vi "check_local_waveform_cache_for_files.vi"() -> ()   [LabVIEW 2013]
uses:
  <vilib>/Utility/miscctls.llb/LVPointTypeDef.ctl
  <userlib>/_OpenG.lib/file/file.llb/Strip Path Extension - Path__ogtk.vi
  <vilib>/addons/database/Connection.llb/Conn Execute.vi
  <vilib>/addons/database/Recordset.llb/Rec Fetch Recordset Data (R).vi
  <vilib>/addons/database/Recordset.llb/Rec Destroy - Connection.vi
  <vilib>/addons/database/_DB Variant To Data/Database Variant To Data.xnode
  <vilib>/addons/database/NI_Database_API.lvlib
panel:
  out "error out":errorcluster
  out "Number of files with no entry":i32
  out "No Database Entry":string[](array[string])
  in  "Run?":bool
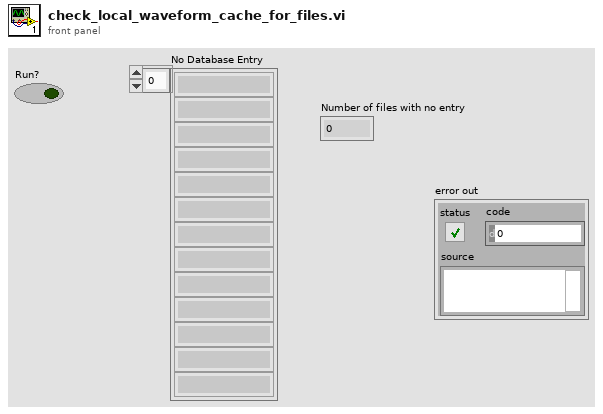
[diagram p1: front panel]
types:
  T1 = typedef "LVPointTypeDef.ctl" = cluster{"Horizontal":i16, "Vertical":i16}
  T2 = typedef "NI_Database_API.lvlib/Conn ObjectReference.ctl" = refnum<k1>
  T3 = typedef "NI_Database_API.lvlib/Rec ObjectReference.ctl" = refnum<k1>
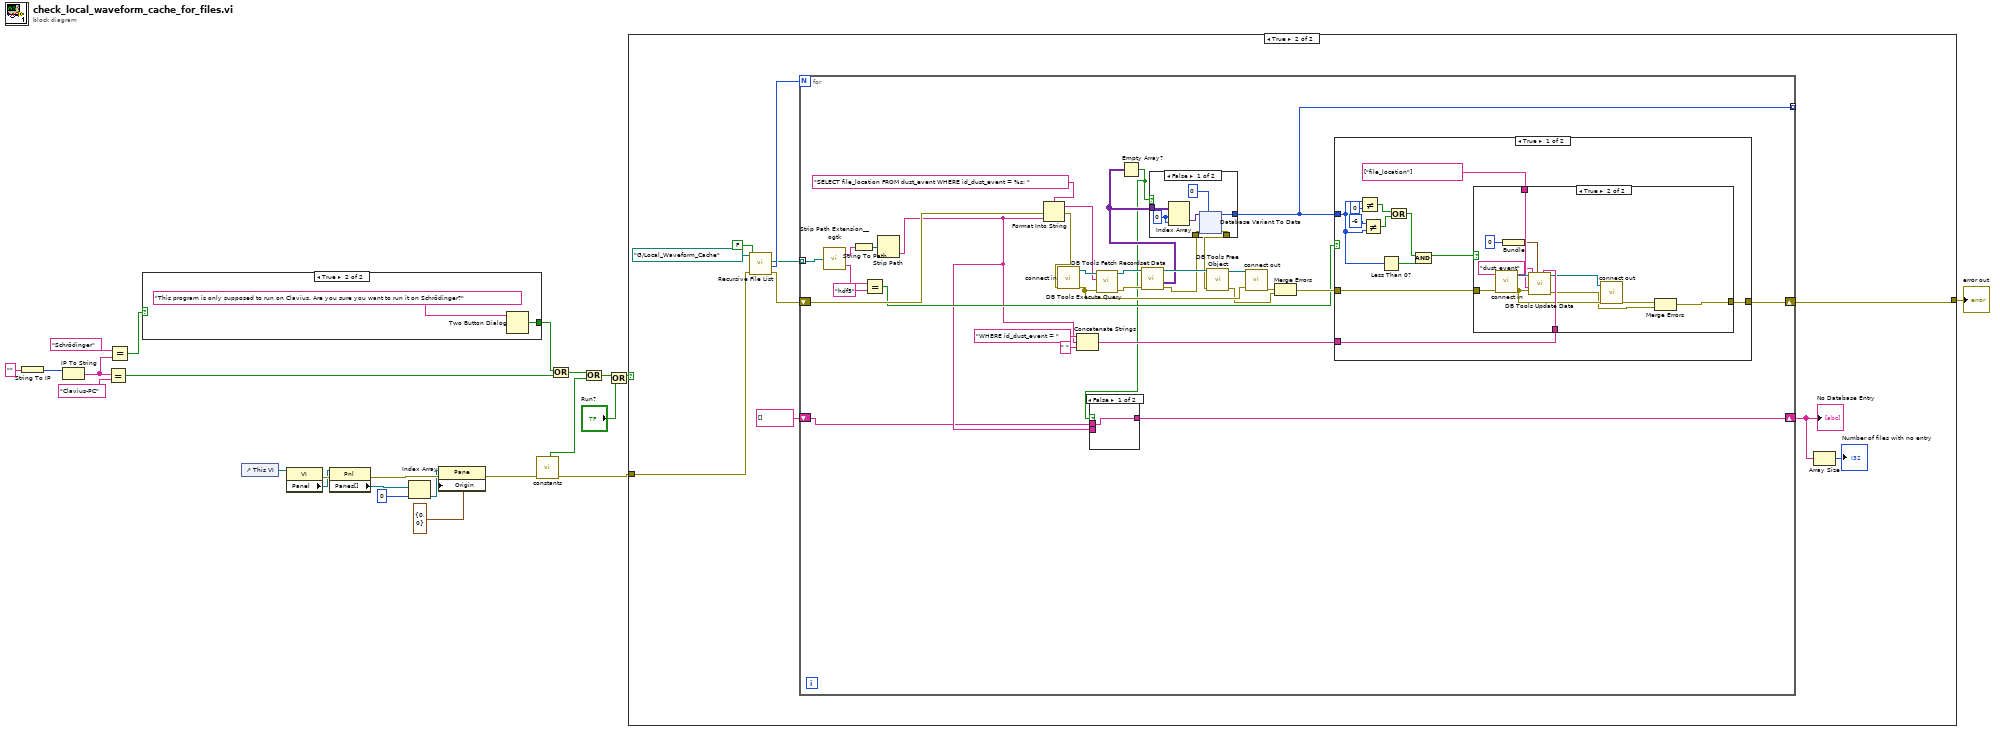
[diagram p0: block diagram]
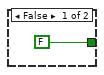
[diagram p2: hidden frame]
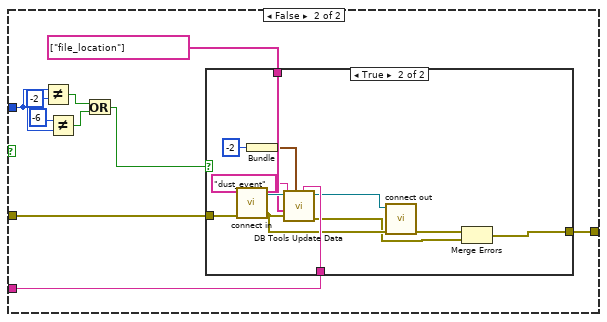
[diagram p5: hidden frame]
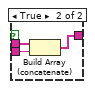
[diagram p7: hidden frame]
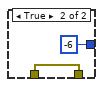
[diagram p8: hidden frame]
diagram:
  n1 = String To IP(1:"" ("name")) -> (0:w16:u32)
  n2 = IP To String(2:w16) -> (0:w11:string)  [unwired: 1 in]
  n3 = Equal?(x=w11, y="Clavius-PC") -> (x = y?=w8:bool)
  n4 = Equal?(x="Schrödinger", y=w11) -> (x = y?=w6:bool)
  n5 = case shown="True" w6 {
    tunnel: [FALSE ("T button?") w27] -> w7
    frame False {
    }
    frame True {
      n6 = Two Button Dialog(message="This program is only supposed to run on Clavius. Are you sure you want to run it on Schrödinger?") -> (T button?=w27:bool)  [unwired: 2 in]
    }
  }
  n7 = control-ref of="This VI"() -> (w24:refnum<vi>)
  n8 = property class="VI"(reference=w24) -> (error out=w23:errorcluster, "Panel"=w22:refnum<vi>)  [unwired: 1 in, 1 out]
  n9 = property class="Pnl"(reference=w22, error in=w23) -> (error out=w21:errorcluster, "Panes[]"=w20:refnum<vi>[])  [unwired: 1 out]
  n10 = Index Array(array=w20, index=0) -> (element=w18:refnum<vi>)
  n11 = property class="Pane"(reference=w18, error in=w21, "Origin"=T1 {"Horizontal"=0, "Vertical"=0}) -> (error out=w13:errorcluster)  [unwired: 1 out]
  n12 = call "constants.vi"("error in (no error)"=w13) -> ("error out"=w4:errorcluster, "Testing"=w12:bool)  [unwired: 4 in, 5 out]
  n13 = Or(x=w7, y=w8) -> (x .or. y?=w9:bool)
  n14 = Or(x=w9, y=w12) -> (x .or. y?=w5:bool)
  n15 = Or(x=w5, y="Run?") -> (x .or. y?=w3:bool)
  n16 = case shown="True" w3 {
    tunnel: w4 -> [w28 w36]
    tunnel: [w28 w29] -> w1
    frame False {
    }
    frame True {
      n17 = call <vilib>:"Recursive File List.vi"("error in (no error)"=w36, "Treat LLBs as Folders?"=FALSE, "Folder Path"=path "G:/Local_Waveform_Cache") -> ("error out"=w33:errorcluster, "Number of Files"=w35:i32, "All Files in Dir"=w34:path[])  [unwired: 4 in, 2 out]
      n18 = for {
        N: w35 -> [_]
        tunnel: w34 -> [w69] mode=indexing
        tunnel: [w45] -> _ mode=indexing
        shift-right: [w42] -> w31
        shift-left: string[] [] -> [w41]
        shift-right: [w39] -> w29
        shift-left: w33 -> [w64]
        n19 = call-poly <userlib>:"Strip Path Extension__ogtk.vi"("path"=w69) -> ("root"=w68:string, "extension"=w66:string)
        n20 = String To Path(string=w68) -> (path=w67:path)
        n21 = Equal?(x=w66, y="hdf5") -> (x = y?=w46:bool)
        n22 = Strip Path(path=w67) -> (name=w43:string)  [unwired: 1 out]
        n23 = Format Into String(format string="SELECT file_location FROM dust_event WHERE id_dust_event = %s; " ("SQL query"), error in=w64, w43) -> (resulting string=w58:string, error out=w59:errorcluster)  [unwired: 1 in]
        n24 = call "connect in.vi"("error in (no error)"=w59) -> ("error out"=w63:errorcluster, "Database Connection"=w61:T2)  [unwired: 6 in, 1 out]
        n25 = Concatenate Strings("WHERE id_dust_event = " ("string"), w43, " " ("string")) -> (w47:string)
        n26 = call-poly <vilib>:"DB Tools Execute Query.vi"("error in (no error)"=w63, "SQL query"=w58, "connection reference"=w61) -> ("error out"=w62:errorcluster, "recordset reference"=w57:T3)  [unwired: 5 in]
        n27 = call-poly <vilib>:"DB Tools Fetch Recordset Data.vi"("error in (no error)"=w62, "recordset reference"=w57) -> ("error out"=w54:errorcluster, "recordset data"=w44:variant[][], "recordset reference out"=w56:T3)  [unwired: 3 in]
        n28 = Empty Array?(array=w44) -> (empty?=w40:bool)
        n29 = case shown="False" w40 {
          tunnel: w43 -> [_ w121]
          tunnel: [w118 w120] -> w42
          tunnel: w41 -> [w118 w119]
          frame False {
          }
          frame True {
            n30 = Build Array (concatenate)(w119, w121) -> (w120:string[])
          }
        }
        n31 = case shown="False" w40 {
          tunnel: w54 -> [w126 w162]
          tunnel: [w125 w162] -> w53
          tunnel: [w123 -6 ("data")] -> w45
          tunnel: w44 -> [w122 _]
          frame False {
            w128 = 0 ("index (row)")
            n32 = Index Array(array=w122, index (row)=w128, index (col)=w128) -> (element=w127:variant)
            n33 = xnode "Database Variant To Data"("database variant"=w127, "error in (no error)"=w126, "type"=0 ("index (row)")) -> ("data"=w123:i32, "error out"=w125:errorcluster)
          }
          frame True {
          }
        }
        n34 = call-poly <vilib>:"DB Tools Free Object.vi"("error in (no error)"=w53, "recordset reference"=w56) -> ("error out"=w51:errorcluster, "connection reference"=w55:T2)  [unwired: 8 in]
        n35 = call "connect out.vi"("error in (no error)"=w63, "connection reference"=w55) -> ("error out"=w52:errorcluster)  [unwired: 9 in]
        n36 = Merge Errors(w52, w51) -> (w50:errorcluster)
        n37 = case shown="True" w46 {
          tunnel: w45 -> [w70 w104]
          tunnel: w50 -> [w77 w99]
          tunnel: w47 -> [w74 w96]
          tunnel: [w73 w95] -> w39
          frame True {
            n38 = Not Equal?(x=w70, y=0) -> (x != y?=w78:bool)
            n39 = Not Equal?(x=-6, y=w70) -> (x != y?=w79:bool)
            n40 = Less Than 0?(x=w70) -> (x < 0?=w71:bool)
            n41 = Or(x=w78, y=w79) -> (x .or. y?=w76:bool)
            n42 = And(x=w76, y=w71) -> (x .and. y?=w72:bool)
            n43 = case shown="True" w72 {
              tunnel: w77 -> [w82 w94]
              tunnel: string[] ["file_location"] ("columns") -> [_ w92]
              tunnel: w74 -> [_ w88]
              tunnel: [w82 w84] -> w73
              frame False {
              }
              frame True {
                n44 = call "connect in.vi"("error in (no error)"=w94) -> ("error out"=w85:errorcluster, "Database Connection"=w93:T2)  [unwired: 6 in, 1 out]
                n45 = Bundle(0) -> (w89:cluster{i32})  [unwired: 1 in]
                n46 = call <vilib>:"DB Tools Update Data.vi"("condition"=w88, "data"=w89, "error in (no error)"=w85, "columns"=w92, "table"="dust_event", "connection reference"=w93) -> ("error out"=w83:errorcluster, "connection reference out"=w87:T2)  [unwired: 4 in]
                n47 = call "connect out.vi"("error in (no error)"=w85, "connection reference"=w87) -> ("error out"=w86:errorcluster)  [unwired: 9 in]
                n48 = Merge Errors(w86, w83) -> (w84:errorcluster)
              }
            }
          }
          frame False {
            n49 = Not Equal?(x=w104, y=-2) -> (x != y?=w100:bool)
            n50 = Not Equal?(x=-6, y=w104) -> (x != y?=w101:bool)
            n51 = Or(x=w100, y=w101) -> (x .or. y?=w98:bool)
            n52 = case shown="True" w98 {
              tunnel: w99 -> [w105 w117]
              tunnel: string[] ["file_location"] ("columns") -> [_ w115]
              tunnel: w96 -> [_ w111]
              tunnel: [w105 w107] -> w95
              frame False {
              }
              frame True {
                n53 = call "connect in.vi"("error in (no error)"=w117) -> ("error out"=w108:errorcluster, "Database Connection"=w116:T2)  [unwired: 6 in, 1 out]
                n54 = Bundle(-2) -> (w112:cluster{i32})  [unwired: 1 in]
                n55 = call <vilib>:"DB Tools Update Data.vi"("condition"=w111, "data"=w112, "error in (no error)"=w108, "columns"=w115, "table"="dust_event", "connection reference"=w116) -> ("error out"=w106:errorcluster, "connection reference out"=w110:T2)  [unwired: 4 in]
                n56 = call "connect out.vi"("error in (no error)"=w108, "connection reference"=w110) -> ("error out"=w109:errorcluster)  [unwired: 9 in]
                n57 = Merge Errors(w109, w106) -> (w107:errorcluster)
              }
            }
          }
        }
      }
      "No Database Entry" <- w31
      n58 = Array Size(array=w31) -> (size(s)=→"Number of files with no entry":i32)
    }
  }
  "error out" <- w1
